vi "Get Artist Names and IDs.vi"(8 "error in (no error)":errorcluster, 11 "SQLite Connection in":refnum<class "Connection.lvclass">) -> (0 "error out":errorcluster, 2 "배열":T1(array[cluster]), 3 "SQLite Connection out":refnum<class "Connection.lvclass">)   [LabVIEW 2015]
doc: "Returns all the artist names and IDs in the database."
uses:
  <vilib>/drjdpowell/SQLite Library/SQL Connection/Connection.lvclass
  <vilib>/drjdpowell/SQLite Library/SQL Statement/SQL Statement.lvclass/SQL Statement.ctl
  <vilib>/drjdpowell/SQLite Library/SQL Statement/Column I64.vi
  <vilib>/drjdpowell/SQLite Library/SQL Statement/Error Message.vi
  <vilib>/drjdpowell/SQLite Library/SQL Statement/Column String.vi
  <vilib>/drjdpowell/SQLite Library/SQL Statement/SQL Statement.lvclass
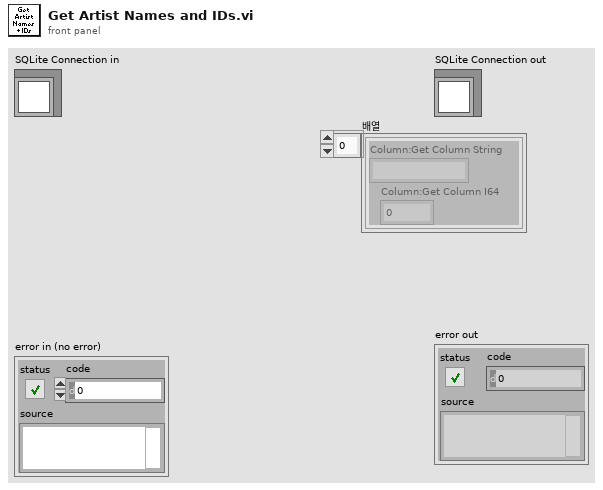
[diagram p1: front panel]
types:
  T1 = cluster{"Column:Get Column String":string, "Column:Get Column I64":i64}[]
  T2 = cluster{"Column:Get Column String":string, "Column:Get Column I64":i64}
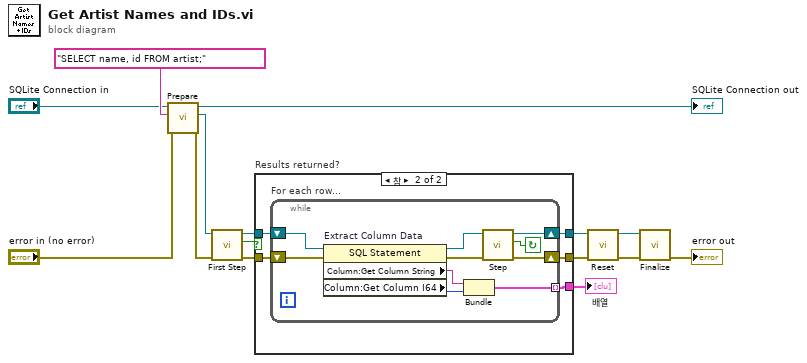
[diagram p0: block diagram]
diagram:
  n1 = call <vilib>:"Prepare.vi"("error in (no error)"="error in (no error)", "SQL"="SELECT name, id FROM artist;", "SQLite Connection in"="SQLite Connection in") -> ("error out"=w6:errorcluster, "SQL Statement"=w7:refnum<class "SQL Statement.lvclass">, "SQLite Connection"=→"SQLite Connection out":refnum<class "Connection.lvclass">)  [unwired: 4 in, 2 out]
  n2 = call <vilib>:"First Step.vi"("error in (no error)"=w6, "SQL Statement in"=w7) -> ("error out"=w14:errorcluster, "Row returned"=w15:bool, "SQL Statement"=w13:refnum<class "SQL Statement.lvclass">)  [unwired: 7 in]
  n3 = case "Results returned?" shown="참" w15 {
    tunnel: [w17 w22] -> w12
    tunnel: [w16 w21] -> w11
    tunnel: w13 -> [w17 w20]
    tunnel: w14 -> [w16 w19]
    tunnel: [_ w18] -> w1
    frame False {
    }
    frame True {
      n4 = while "For each row..." {
        shift-right: [w31] -> w22
        shift-left: w20 -> [w28]
        shift-right: [w29] -> w21
        shift-left: w19 -> [w27]
        tunnel: [w24] -> w18 mode=indexing
        stop <- w26 continue-if-true
        n5 = property on="Extract Column Data" class="SQL Statement"(reference=w28, error in=w27) -> (reference out=w32:refnum<class "SQL Statement.lvclass">, error out=w30:errorcluster, "Column:Get Column String"=w23:string, "Column:Get Column I64"=w25:i64)
        n6 = Bundle("Column:Get Column String"=w23, "Column:Get Column I64"=w25) -> (w24:T2)  [unwired: 1 in]
        n7 = call <vilib>:"Step.vi"("error in (no error)"=w30, "SQL Statement in"=w32) -> ("error out"=w29:errorcluster, "Row returned"=w26:bool, "SQL Statement"=w31:refnum<class "SQL Statement.lvclass">)  [unwired: 7 in]
      }
    }
  }
  "배열" <- w1
  n8 = call <vilib>:"Reset.vi"("error in (no error)"=w11, "SQL Statement in"=w12) -> ("error out"=w4:errorcluster, "SQL Statement"=w5:refnum<class "SQL Statement.lvclass">)  [unwired: 8 in]
  n9 = call <vilib>:"Finalize.vi"("error in (no error)"=w4, "SQL Statement in"=w5) -> ("error out"=→"error out":errorcluster)  [unwired: 9 in]
